vi "Intake_TEST.vi"(11 "CLUSTERIN":T1) -> (3 "ClusterOUT":T1)   [LabVIEW 2018]
uses:
  TypeDefs/Teleop Data Cluster.ctl
  TypeDefs/Joystick Buttons.ctl
  TypeDefs/Joystick Axes.ctl
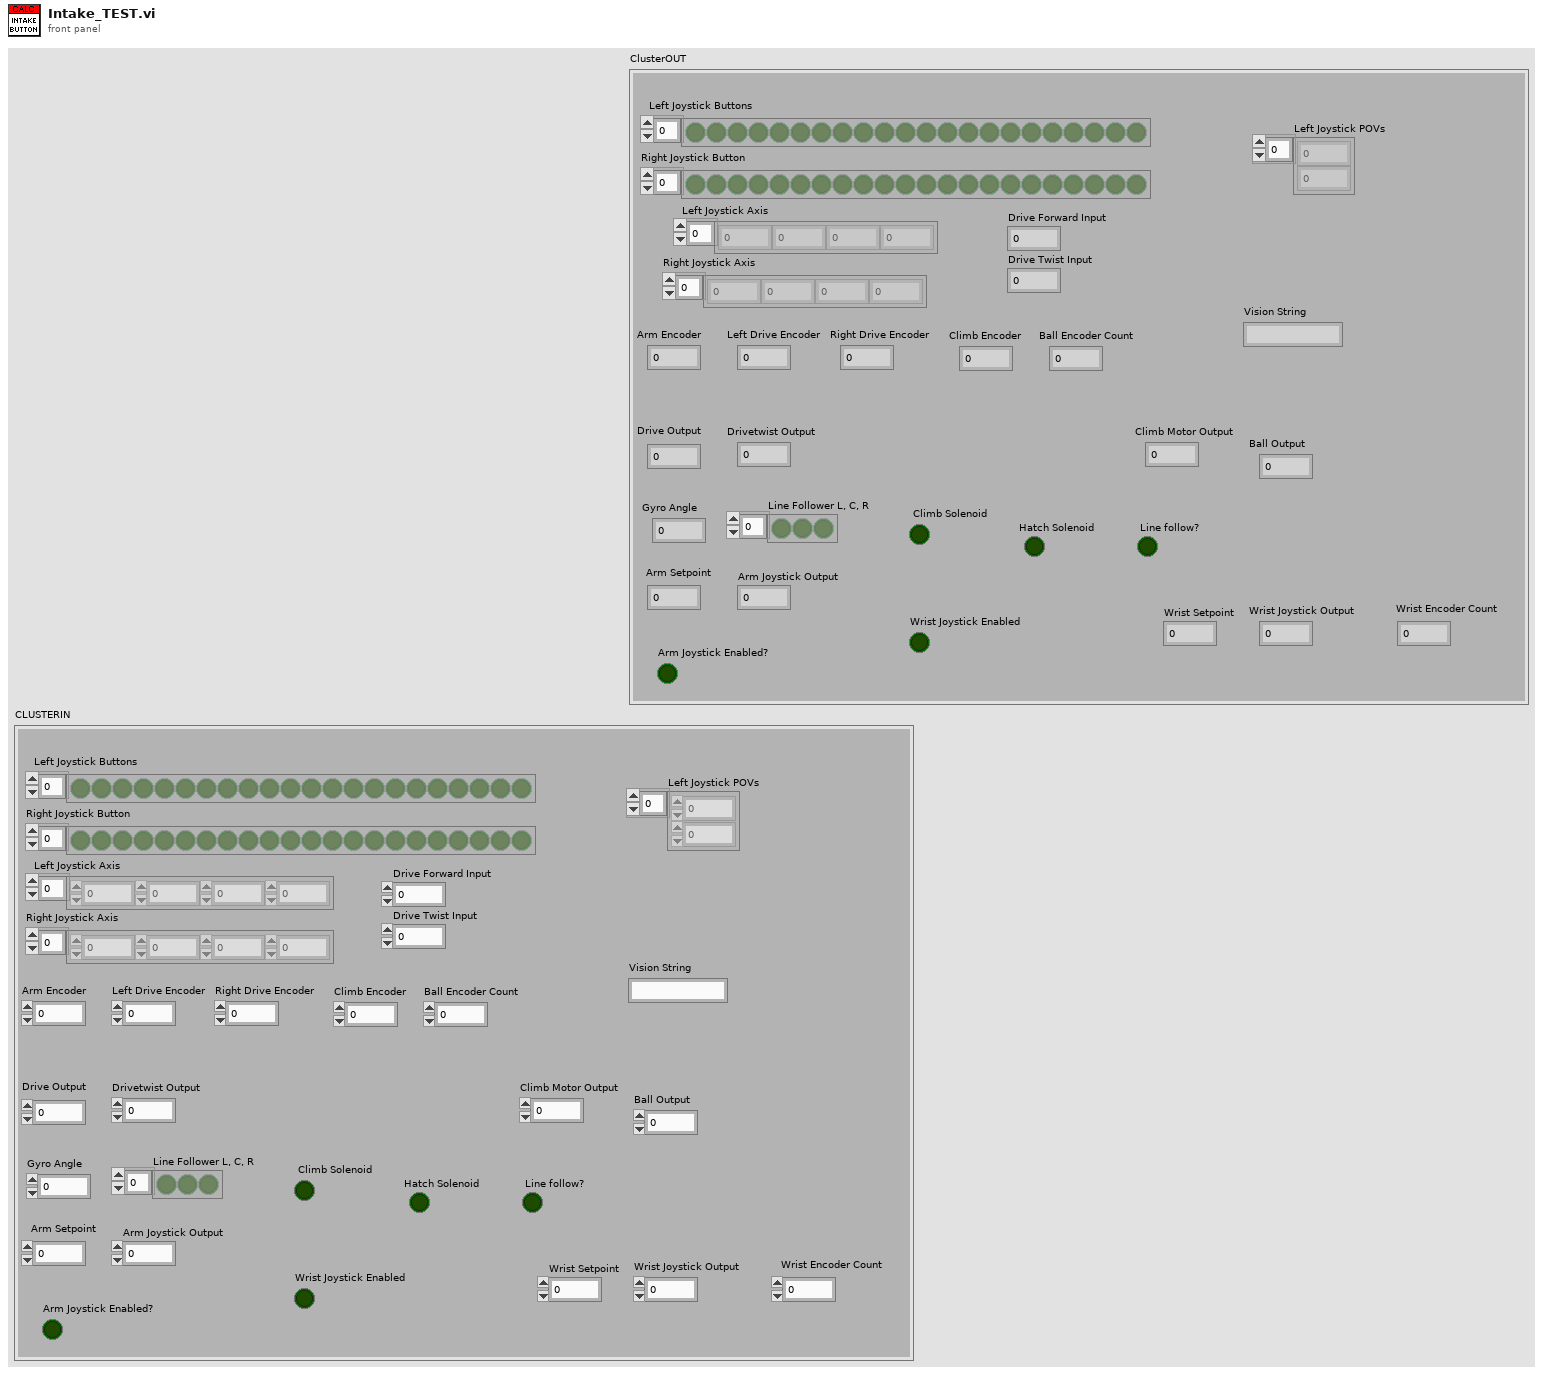
[diagram p1: front panel]
types:
  T1 = typedef "Teleop Data Cluster.ctl" = cluster{"Drive Forward Input ":dbl, "Drive Twist Input":dbl, "Drive Output":dbl, "Drivetwist Output":dbl, "Left Joystick Buttons":bool[], "Left Joystick Axis":dbl[], "Right Joystick Axis":dbl[], "Right Joystick Button":bool[], "Arm Encoder":dbl, "Left Drive Encoder":dbl, "Right Drive Encoder":dbl, "Gyro Angle ":dbl, "Arm Joystick Output  ":dbl, "Line Follower L, C, R ":bool[], "Line follow?":bool, " Climb Solenoid":bool, "Wrist Encoder Count":dbl, "Wrist Joystick Output":dbl, "Ball Encoder Count":dbl, "Ball Output":dbl, "Climb Encoder":dbl, "Climb Motor Output":dbl, " Hatch Solenoid":bool, "Arm Setpoint ":dbl, "Wrist Setpoint ":dbl, "Arm Joystick Enabled?":bool, "Wrist Joystick Enabled":bool, "Vision String":string, "Left Joystick POVs":i16[]}
  T2 = typedef "Joystick Axes.ctl" = enum16{"X Axis", "Y Axis", "Twist Axis", "Throttle"}
  T3 = typedef "Joystick Buttons.ctl" = enum16{"Trigger", "Thumb", "Top 3", "Top 4", "Top 5", "Top 6", "Bottom 7", "Bottom 8", "Bottom 9", "Bottom 10", "Bottom 11", "Bottom 12"}
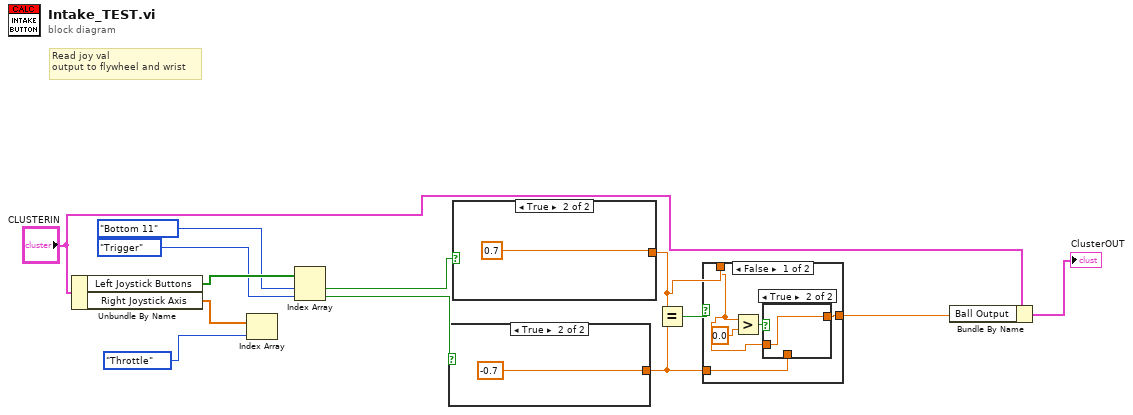
[diagram p0: block diagram]
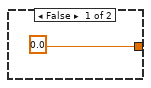
[diagram p4: hidden frame]
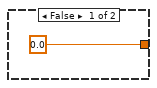
[diagram p5: hidden frame]
diagram:
  # "Read joy val\noutput to flywheel and wrist"
  n1 = Unbundle By Name("CLUSTERIN") -> ("Left Joystick Buttons"=w13:bool[], "Right Joystick Axis"=w3:dbl[])
  n2 = Index Array(array=w3, index=Joystick_Axes."Throttle" ("Enum")) -> ()  [unwired: 1 out]
  n3 = Index Array(array=w13, index #1=Joystick_Buttons."Bottom 11" ("Enum"), index #2=Joystick_Buttons."Trigger" ("Enum")) -> (element #1=w10:bool, element #2=w9:bool)
  n4 = case shown="True" w9 {
    tunnel: [0.0 -0.7] -> w6
    frame False {
    }
    frame True {
    }
  }
  n5 = case shown="True" w10 {
    tunnel: [0.0 0.7] -> w7
    frame False {
    }
    frame True {
    }
  }
  n6 = Equal?(x=w7, y=w6) -> (x = y?=w4:bool)
  n7 = case shown="False" w4 {
    tunnel: [w19 w25] -> w8
    tunnel: w7 -> [w20 w25]
    tunnel: w6 -> [w18 _]
    frame False {
      n8 = Greater?(x=w20, y=0.0) -> (0:w21:bool)
      n9 = case shown="True" w21 {
        tunnel: w20 -> [_ w24]
        tunnel: [w23 w24] -> w19
        tunnel: w18 -> [w23 _]
        frame False {
        }
        frame True {
        }
      }
    }
    frame True {
    }
  }
  n10 = Bundle By Name(cluster="CLUSTERIN", "Ball Output"=w8) -> (→"ClusterOUT":T1)
